vi "StartApp Event.vi"(8 "error in (no error)":errorcluster, 9 "Source":T1, 11 "EventLog in":refnum<class "EventLog.lvclass">) -> (0 "error out":errorcluster, 3 "Events out":refnum<class "Event.lvclass">)   [LabVIEW 2019, in "Event.lvclass"]
uses:
  Event.lvclass
  SubModules/EventLog/EventLog.lvclass
  TypeDef/Event Classification.ctl
  SubModules/LogsAbstract/TypeDef/Event Source.ctl
  SubModules/LogsAbstract/LogsAbstract.lvclass
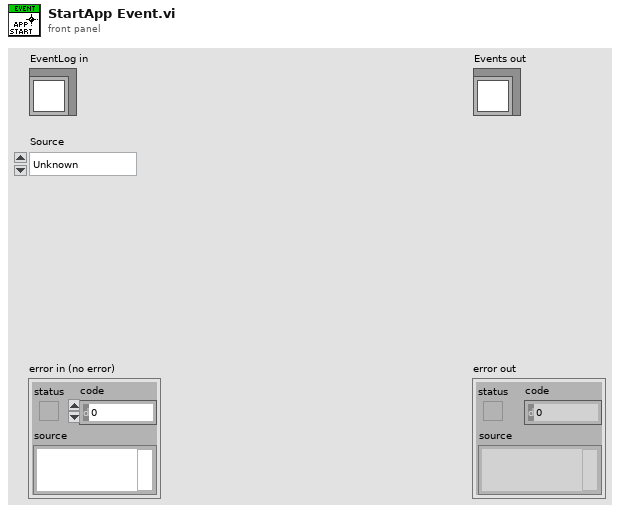
[diagram p1: front panel]
types:
  T1 = typedef "LogsAbstract.lvlib/LogsAbstract.lvclass/Event Source.ctl" = enum16{"Unknown", "< --- Modules --- >", "Core", "< --- SubModules --- >", "Core -> EventLog", "Core -> ErrorLog"}
  T2 = typedef "Event.lvclass/Event Classification.ctl" = enum16{"System Log", "test1", "test2", "test3"}
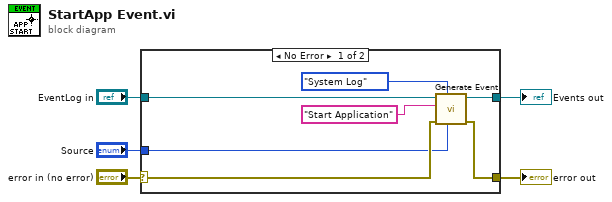
[diagram p0: block diagram]
diagram:
  n1 = case shown="No Error" "error in (no error)" {
    selector: "error in (no error)" -> [w10 w13]
    tunnel: [w9 w13] -> w4
    tunnel: [w12 _] -> w3
    tunnel: "EventLog in" -> [w8 _]
    tunnel: "Source" -> [w6 _]
    frame No Error {
      n2 = call "Generate Event.vi"("Source"=w6, "Classification"=Event_Classification."System Log", "Error In"=w10, "Description"="Start Application", "EventLog in"=w8) -> ("Error Out"=w9:errorcluster, "Events out"=w12:refnum<class "Event.lvclass">)  [unwired: 5 in]
    }
    frame Error {
    }
  }
  "error out" <- w4
  "Events out" <- w3
